vi "Proximity sensors - MAIN.vi"() -> ()   [LabVIEW 2022 SP3]
uses:
  States.ctl
  Main cluster.ctl
  <vilib>/Utility/file.llb/Write Delimited Spreadsheet (DBL).vi
  <vilib>/gmath/NI_Gmath.lvlib
panel:
  out "Distance Bar":dbl(slide) scale=15.0..180.0
  out "Distance (cm)":dbl format="%#_3g"
  out "Voltage":dbl format="%#_2g"
  in  "Select sensor":enum16{"Ultrasonic", "IR"}(ring)
  out "Alarm":bool
  out "Waveform Chart":cluster{"Numeric":dbl, "Scalar":dbl}(graph)
  in  "Interpolation method":T1(ring)=enum."linear"
  in  "Finish measurement":bool
  in  "Save Button":bool
  in  "Calibration":bool
  in  "Measurement":bool
  in  "Stop Button":bool
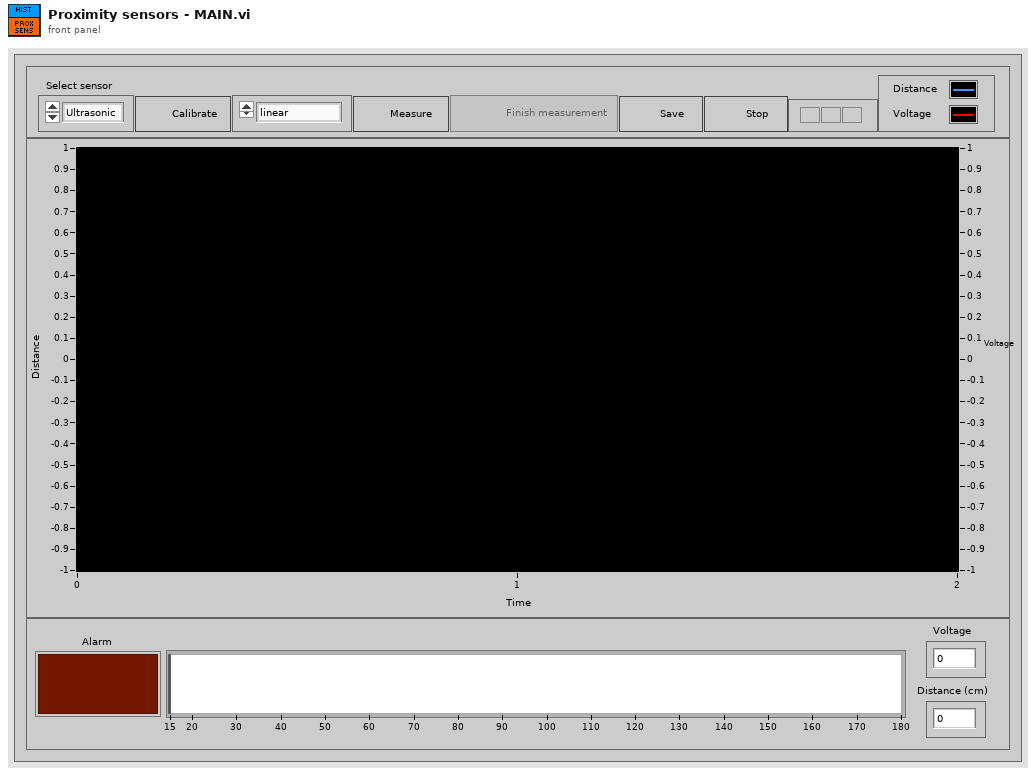
[diagram p1: front panel]
types:
  T1 = enum16{"nearest", "linear", "spline", "cubic Hermite", "Lagrange"}
  T2 = typedef "Main cluster.ctl" = cluster{"Distance [cm]| Voltage [V]":dbl[][], "Measured distance":dbl[]}
  T3 = typedef "States.ctl" = enum16{"Initialize", "Wait for Event", "Calibrate", "Measure", "Save", "Stop"}
  T4 = enum8{"Enabled", "Disabled", "Disabled and Grayed Out"}
  T5 = cluster{"Distance [cm]| Voltage [V]":dbl[][], "Measured distance":dbl[]}
  T6 = cluster{"Distance [cm]| Voltage [V]":dbl[][], dbl[]}
  T7 = typedef "imagedata.ctl" = cluster{"image type":i32, "image depth":i32, "image":u8[], "mask":u8[], "colors":u32[], "Rectangle":cluster{"left":i16, "top":i16, "right":i16, "bottom":i16}}
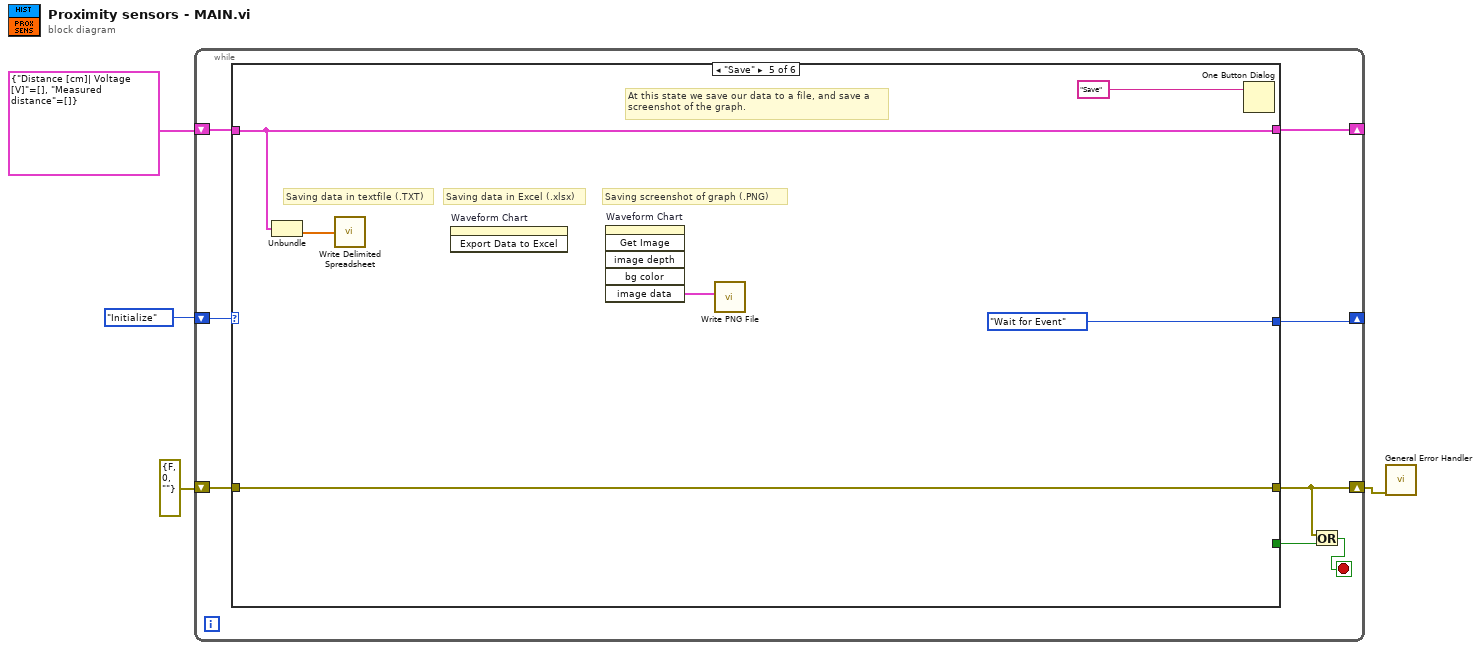
[diagram p0: block diagram]
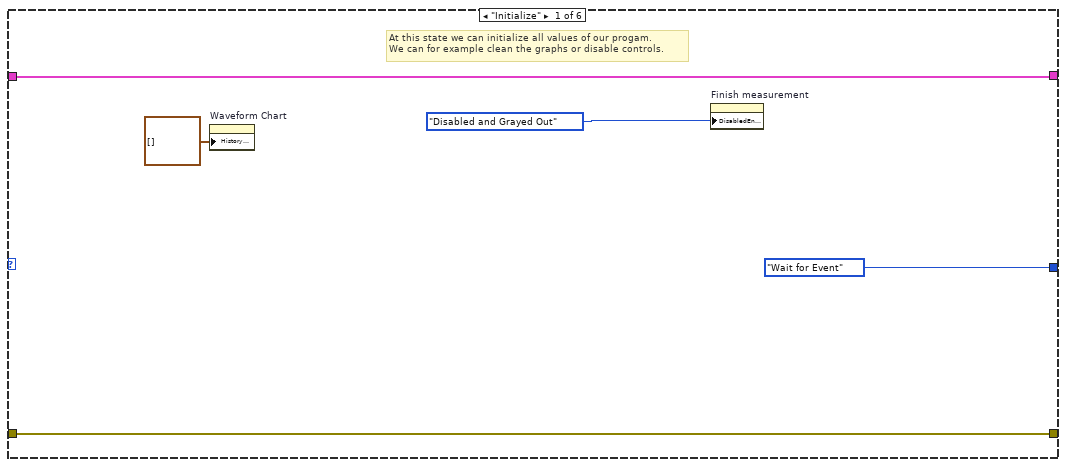
[diagram p2: hidden frame]
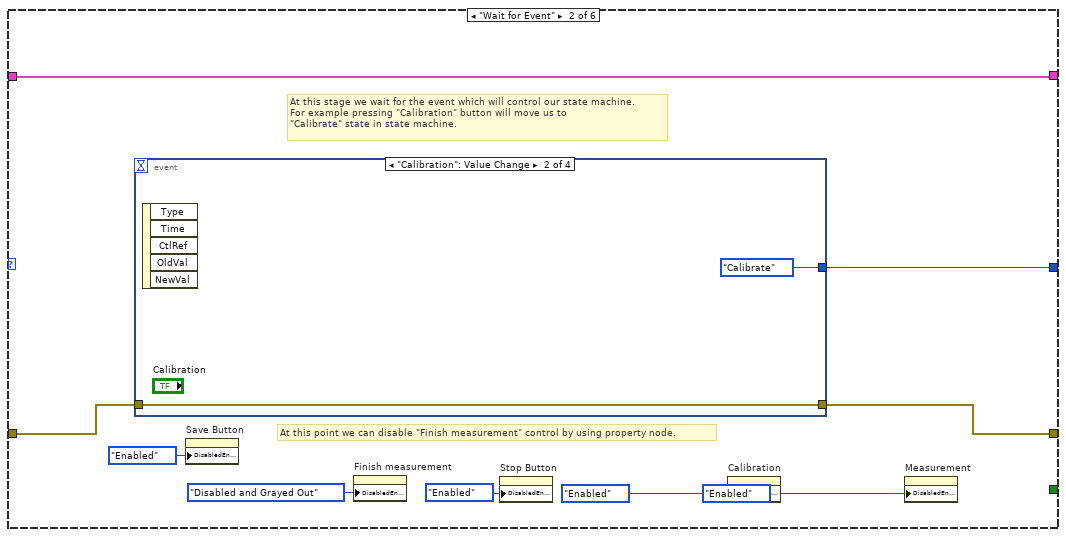
[diagram p3: hidden frame]
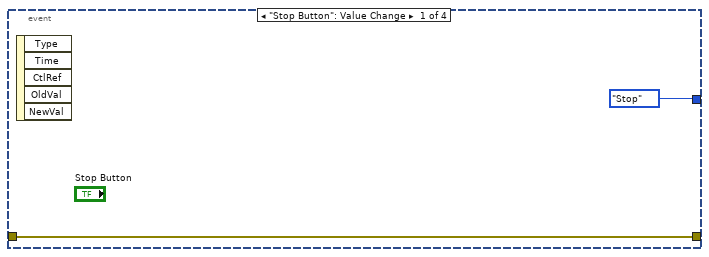
[diagram p4: hidden frame]
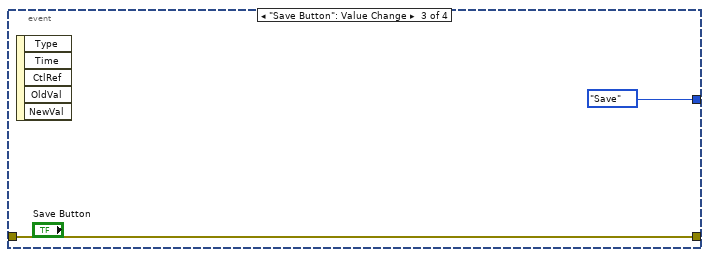
[diagram p5: hidden frame]
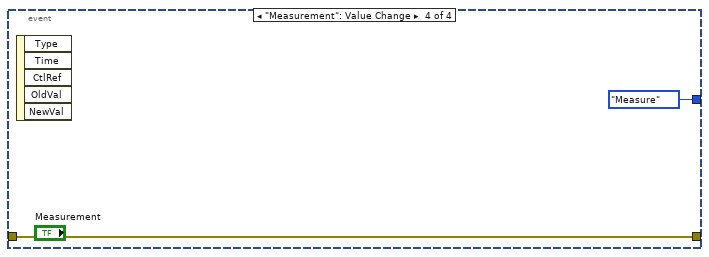
[diagram p6: hidden frame]
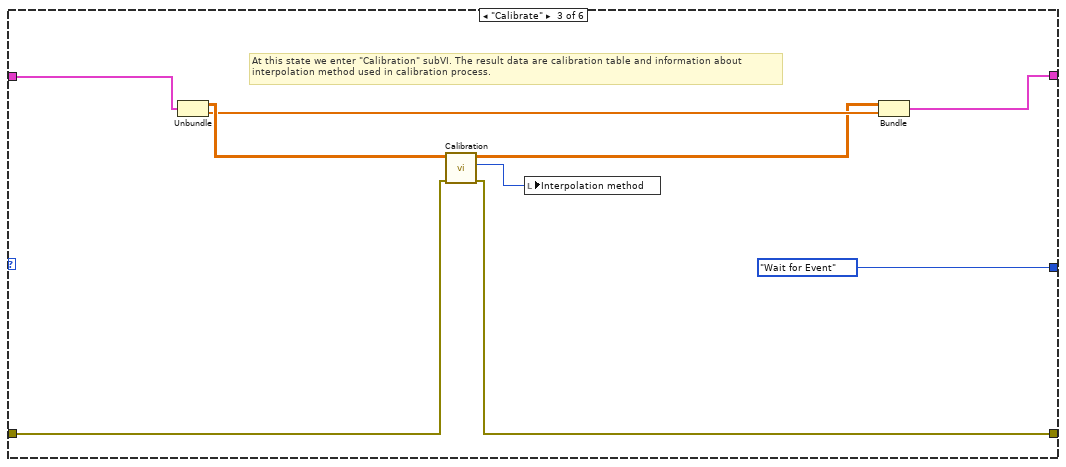
[diagram p7: hidden frame]
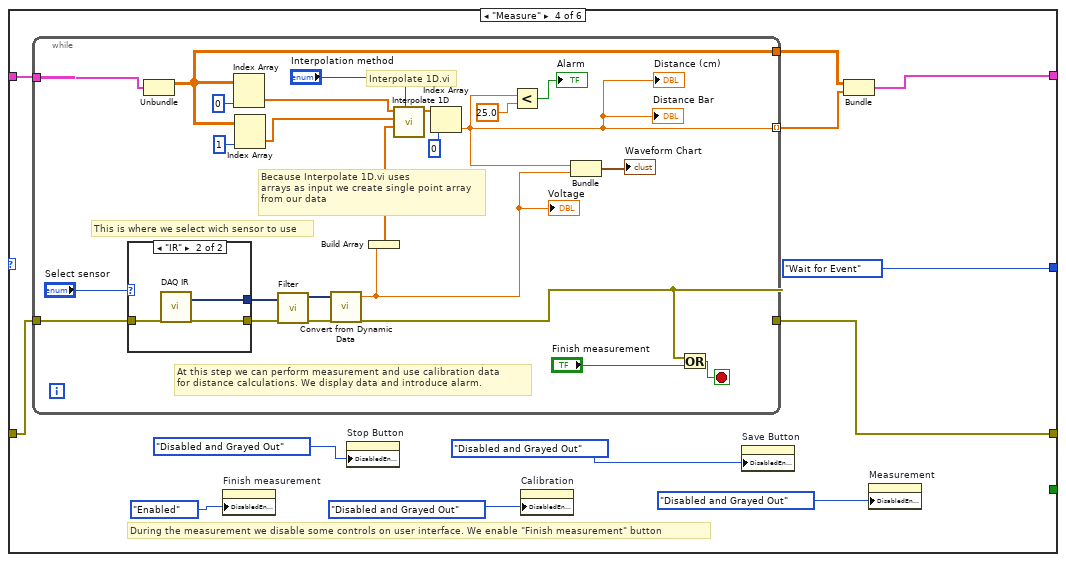
[diagram p8: hidden frame]
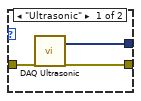
[diagram p9: hidden frame]
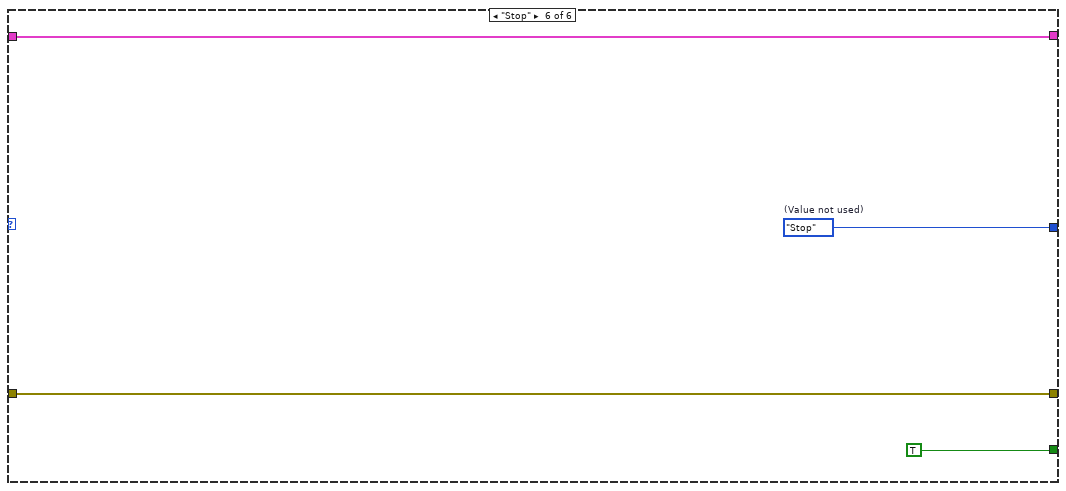
[diagram p10: hidden frame]
diagram:
  n1 = while {
    shift-right: [w11] -> _
    shift-left: States."Initialize" -> [w12]
    shift-right: [w8] -> w2
    shift-left: errorcluster {"status"=FALSE, "code"=0, "source"=""} ("error constant") -> [w10]
    shift-right: [w5] -> _
    shift-left: T2 {"Distance [cm]| Voltage [V]"=[], "Measured distance"=[]} ("Main cluster") -> [w6]
    stop <- w7 stop-if-true
    n2 = case shown="\"Save\"" w12 {
      tunnel: [States."Wait for Event" w26 States."Wait for Event" States."Wait for Event" States."Wait for Event" w93] -> w11
      tunnel: [_ _ _ _ _ TRUE] -> w9
      tunnel: w10 -> [w16 w25 w42 w53 w89 w92]
      tunnel: [w16 w24 w41 w52 w89 w92] -> w8
      tunnel: [w13 w18 w35 w44 w87 w91] -> w5
      tunnel: w6 -> [w13 w18 w39 w47 w87 w91]
      frame "Initialize" {
        # "At this state we can initialize all values of our progam.\nWe can for example clean the graphs or disable controls."
        n3 = property on="Waveform Chart" class="WFChart (strict)"("History Data"=cluster{"Numeric":dbl, "Scalar":dbl}[] []) -> ()  [unwired: 2 in, 2 out]
        n4 = property on="Finish measurement" class="Bool"("DisabledEnum"=T4."Disabled and Grayed Out" ("Disabled")) -> ()  [unwired: 2 in, 2 out]
      }
      frame "Wait for Event" {
        # "At this point we can disable \"Finish measurement\" control by using property node."
        # "At this stage we wait for the event which will control our state machine.\nFor example pressing \"Calibration\" button will move us to \n\"Calibrate\" state in state machine."
        n5 = event shown="[1] \"Calibration\": Value Change" {
          selector: _ -> [_ _ _ _]
          dyn-events: _ -> [_ _ _ _]
          timeout: _ -> [_ _ _ _]
          tunnel: [States."Stop" States."Calibrate" States."Save" States."Measure"] -> w26
          tunnel: w25 -> [w27 w30 w31 w34]
          tunnel: [w27 w30 w31 w34] -> w24
          event "Stop Button": Value Change {
            n6 = event-data() -> ()  [unwired: 1 in, 5 out]
          }
          event "Calibration": Value Change {
            n7 = event-data() -> ()  [unwired: 1 in, 5 out]
          }
          event "Save Button": Value Change {
            n8 = event-data() -> ()  [unwired: 1 in, 5 out]
          }
          event "Measurement": Value Change {
            n9 = event-data() -> ()  [unwired: 1 in, 5 out]
          }
        }
        n10 = property on="Save Button" class="Bool"("DisabledEnum"=T4."Enabled" ("Disabled")) -> ()  [unwired: 2 in, 2 out]
        n11 = property on="Finish measurement" class="Bool"("DisabledEnum"=T4."Disabled and Grayed Out" ("Disabled")) -> ()  [unwired: 2 in, 2 out]
        n12 = property on="Stop Button" class="Bool"("DisabledEnum"=T4."Enabled" ("Disabled")) -> ()  [unwired: 2 in, 2 out]
        n13 = property on="Calibration" class="Bool"("DisabledEnum"=T4."Enabled" ("Disabled")) -> ()  [unwired: 2 in, 2 out]
        n14 = property on="Measurement" class="Bool"("DisabledEnum"=T4."Enabled" ("Disabled")) -> ()  [unwired: 2 in, 2 out]
      }
      frame "Calibrate" {
        # "At this state we enter \"Calibration\" subVI. The result data are calibration table and information about \ninterpolation method used in calibration process."
        n15 = Unbundle(w39) -> ("Distance [cm]| Voltage [V]"=w38:dbl[][], "Measured distance"=w37:dbl[])
        n16 = call "Calibration.vi"("error in (no error)"=w42, "Distance [cm]| Voltage [V]"=w38) -> ("error out"=w41:errorcluster, "Interpolation method"=w40:T1, "Distance [cm]| Voltage [V]"=w36:dbl[][])  [unwired: 7 in]
        n17 = local write "Interpolation method"(w40) -> ()
        n18 = Bundle("Distance [cm]| Voltage [V]"=w36, "Measured distance"=w37) -> (w35:T5)  [unwired: 1 in]
      }
      frame "Measure" {
        # "During the measurement we disable some controls on user interface. We enable \"Finish measurement\" button"
        n19 = while {
          tunnel: w53 -> [w65]
          tunnel: [w62] -> w52
          tunnel: [w58] -> w46 mode=indexing
          tunnel: w47 -> [w67]
          tunnel: [w66] -> w45
          stop <- w69 stop-if-true
          # "This is where we select wich sensor to use"
          # "Because Interpolate 1D.vi uses \narrays as input we create single point array\nfrom our data"
          # "Interpolate 1D.vi"
          # "At this step we can perform measurement and use calibration data \nfor distance calculations. We display data and introduce alarm."
          n20 = case shown="\"IR\"" "Select sensor" {
            tunnel: w65 -> [w81 w84]
            tunnel: [w79 w83] -> w64
            tunnel: [w80 w82] -> w61
            frame "Ultrasonic" {
              n21 = call "DAQ Ultrasonic"("error in"=w81) -> ("data"=w80:dynamicdata, "error out"=w79:errorcluster)  [unwired: 15 in, 2 out]
            }
            frame "IR" {
              n22 = call "DAQ IR"("error in"=w84) -> ("data"=w82:dynamicdata, "error out"=w83:errorcluster)  [unwired: 15 in, 2 out]
            }
          }
          n23 = Unbundle(w67) -> ("Distance [cm]| Voltage [V]"=w66:dbl[][])  [unwired: 1 out]
          n24 = Index Array(array=w66, index (col)=0 ("disabled index (col)")) -> (element=w76:dbl[])  [unwired: 1 in]
          n25 = Index Array(array=w66, index (col)=1 ("disabled index (col)")) -> (element=w75:dbl[])  [unwired: 1 in]
          n26 = call "Filter"("error in (no error)"=w64, "Signal"=w61) -> ("error out"=w62:errorcluster, "Filtered Signal"=w63:dynamicdata)  [unwired: 8 in]
          n27 = call "Convert from Dynamic Data"("Dynamic Data Type"=w63) -> ("Scalar"=w59:dbl)  [unwired: 3 in]
          "Voltage" <- w59
          n28 = Build Array(w59) -> (w73:dbl[])
          n29 = call <vilib>:"Interpolate 1D.vi"("method"="Interpolation method", "xi"=w73, "X"=w75, "Y"=w76) -> ("yi"=w72:dbl[])  [unwired: 5 in, 2 out]
          n30 = Index Array(array=w72, index=0) -> (element=w58:dbl)
          "Distance (cm)" <- w58
          "Distance Bar" <- w58
          n31 = Less?(x=w58, y=25.0) -> (x < y?=→"Alarm":bool)
          n32 = Bundle("Numeric"=w58, "Scalar"=w59) -> (→"Waveform Chart":cluster{"Numeric":dbl, "Scalar":dbl})  [unwired: 1 in]
          n33 = Or(x=w62, y="Finish measurement") -> (x .or. y?=w69:bool)
        }
        n34 = property on="Finish measurement" class="Bool"("DisabledEnum"=T4."Enabled" ("Disabled")) -> ()  [unwired: 2 in, 2 out]
        n35 = property on="Stop Button" class="Bool"("DisabledEnum"=T4."Disabled and Grayed Out" ("Disabled")) -> ()  [unwired: 2 in, 2 out]
        n36 = property on="Calibration" class="Bool"("DisabledEnum"=T4."Disabled and Grayed Out" ("Disabled")) -> ()  [unwired: 2 in, 2 out]
        n37 = property on="Save Button" class="Bool"("DisabledEnum"=T4."Disabled and Grayed Out" ("Disabled")) -> ()  [unwired: 2 in, 2 out]
        n38 = Bundle("Distance [cm]| Voltage [V]"=w45, w46) -> (w44:T6)  [unwired: 1 in]
        n39 = property on="Measurement" class="Bool"("DisabledEnum"=T4."Disabled and Grayed Out" ("Disabled")) -> ()  [unwired: 2 in, 2 out]
      }
      frame "Save" {
        # "Saving data in Excel (.xlsx)"
        # "Saving data in textfile (.TXT)"
        # "At this state we save our data to a file, and save a \nscreenshot of the graph."
        # "Saving screenshot of graph (.PNG)"
        n40 = Unbundle(w87) -> ("Measured distance"=w86:dbl[])  [unwired: 1 out]
        n41 = call-poly <vilib>:"Write Delimited Spreadsheet.vi"("1D data"=w86) -> ()  [unwired: 13 in, 2 out]
        n42 = invoke on="Waveform Chart" class="WFChart (strict)" method="Export Data to Excel"() -> ()  [unwired: 3 in, 3 out]
        n43 = invoke on="Waveform Chart" class="WFChart (strict)" method="Get Image"() -> ("image data"=w85:T7)  [unwired: 6 in, 5 out]
        n44 = call <vilib>:"Write PNG File.vi"("image data"=w85) -> ()  [unwired: 9 in, 2 out]
        n45 = One Button Dialog(message="Save") -> ()  [unwired: 1 in, 1 out]
      }
      frame "Stop" {
        w93 = States."Stop"  # (Value not used)
      }
    }
    n46 = Or(x=w8, y=w9) -> (x .or. y?=w7:bool)
  }
  n47 = call <vilib>:"General Error Handler.vi"("error in (no error)"=w2) -> ()  [unwired: 10 in, 5 out]
